vi "YokogawaInputTest.vi"() -> ()   [LabVIEW 2020]
doc: "This example shows how to measure the integrate data."
uses:
  <instrlib>/Yokogawa WT300 Series/Public/Utility/Function/Create Function String (Voltage).vi
  <instrlib>/Yokogawa WT300 Series/Public/Utility/Function/Create Function String (Current).vi
  <instrlib>/Yokogawa WT300 Series/Public/Utility/Function/Create Function String (Power).vi
  <instrlib>/Yokogawa WT300 Series/Public/Utility/Function/Create Function String (Integrate).vi
  <instrlib>/Yokogawa WT300 Series/Public/Utility/Function/Create Function String (Harmonics).vi
  <instrlib>/Yokogawa WT300 Series/Public/Data/Read Measurement (Normal).vi
  <instrlib>/Yokogawa WT300 Series/Yokogawa WT300 Series.lvlib
panel:
  out "Loop Time":u32
  in  "Reset":bool
  out "Function":string[](array[string])
  out "Measurement":dbl[](array[numeric])
  in  "Stop":bool
  in  "Update Rate (100ms)":dbl(ring)=0.1 items=["100m"=0.1, "250m"=0.25, "500m"=0.5, "1"=1.0, "2"=2.0, "5"=5.0]
  in  "Timeout (10000 ms)":i32=10000 min=1
  in  "VISA resource name":refnum<visa-resource-name>="TCPIP::192.168.1.18::INSTR"
  # "(c) 2013 Yokogawa Meters & Instruments Corporation.  All rights reserved."
  # "WT300 SERIES POWER ANALYZER"
  # "s"
  # "ms"
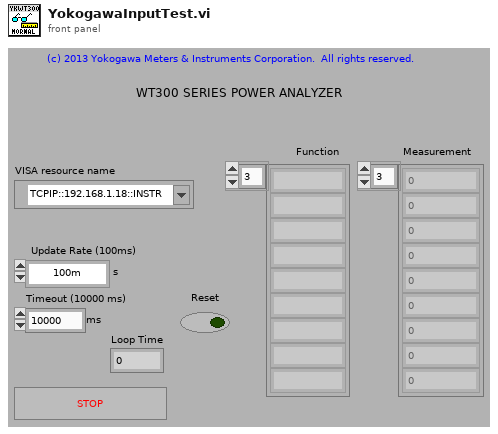
[diagram p1: front panel]
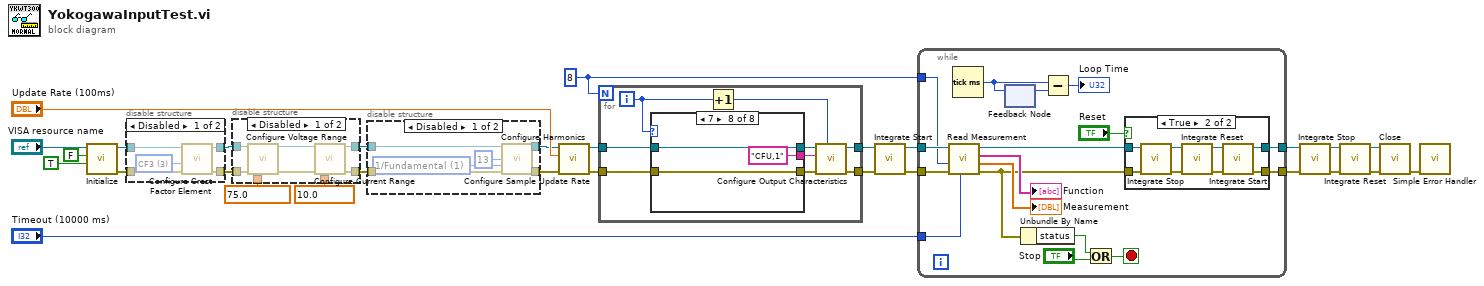
[diagram p0: block diagram]
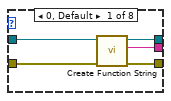
[diagram p5: hidden frame]
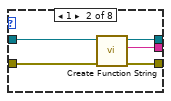
[diagram p6: hidden frame]
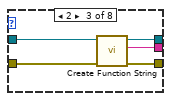
[diagram p7: hidden frame]
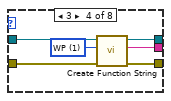
[diagram p8: hidden frame]
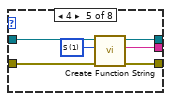
[diagram p9: hidden frame]
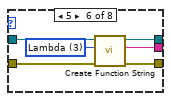
[diagram p10: hidden frame]
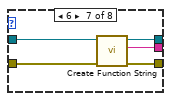
[diagram p11: hidden frame]
diagram:
  w9 = 75.0 items=["15 <7.5>"=7.5, "30 <15>"=15.0, "60 <30>"=30.0, "150 <75>"=75.0, "300 <150>"=150.0, "600 <300>"=300.0] ("Manual Range (600 <300> V)")
  w10 = 10.0 items=["5m <2.5m>"=0.0025, "10m <5m>"=0.005, "20m <10m>"=0.01, "50m <25m>"=0.025, "100m <50m>"=0.05, "200m <100m>"=0.1, "500m <250m>"=0.25, "1 <500m>"=0.5, "2 <1>"=1.0, "5 <2.5>"=2.5, "10 <5>"=5.0, "20 <10>"=10.0, "40 <20>"=20.0] ("Manual Range (20 <10> A)")
  w24 = 8
  n1 = call <instrlib>:"Initialize.vi"("Reset (True)"=TRUE ("Reset? (True)"), "ID Query (True)"=FALSE, "VISA resource name"="VISA resource name") -> ("error out"=w1:errorcluster, "VISA resource name out"=w2:refnum<visa-resource-name>)  [unwired: 7 in]
  n2 = disable-structure shown="Disabled" {
    disable-tunnel: [w34 w36] -> w11
    disable-tunnel: w2 -> [w32 w36]
    disable-tunnel: [w31 w35] -> w8
    disable-tunnel: w1 -> [w30 w35]
    frame Disabled {
      w33 = 3 items=["CF3"=3, "CF6"=6] ("Crest Factor (3: CF3)")
      n3 = call "Configure Crest Factor Element.vi"("error in (no error)"=w30, "Crest Factor (3: CF3)"=w33, "VISA resource name"=w32) -> ("error out"=w31:errorcluster, "VISA resource name out"=w34:refnum<visa-resource-name>)  [unwired: 7 in]
    }
    frame Enabled {
    }
  }
  n4 = disable-structure shown="Disabled" {
    disable-tunnel: w11 -> [w44 w46]
    disable-tunnel: w10 -> [w42 _]
    disable-tunnel: w9 -> [w41 _]
    disable-tunnel: [w40 w46] -> w6
    disable-tunnel: w8 -> [w39 w45]
    disable-tunnel: [w37 w45] -> w4
    frame Disabled {
      n5 = call "Configure Voltage Range.vi"("VISA resource name"=w44, "error in (no error)"=w39, "Manual Range (600 <300> V)"=w41) -> ("VISA resource name out"=w43:refnum<visa-resource-name>, "error out"=w38:errorcluster)  [unwired: 11 in]
      n6 = call "Configure Current Range.vi"("VISA resource name"=w43, "error in (no error)"=w38, "Manual Range (20 <10> A)"=w42) -> ("VISA resource name out"=w40:refnum<visa-resource-name>, "error out"=w37:errorcluster)  [unwired: 11 in]
    }
    frame Enabled {
    }
  }
  n7 = disable-structure shown="Disabled" {
    disable-tunnel: [w50 w54] -> w7
    disable-tunnel: w6 -> [w49 w54]
    disable-tunnel: [w48 w53] -> w5
    disable-tunnel: w4 -> [w47 w53]
    frame Disabled {
      w52 = 1 items=["1/Total", "1/Fundamental"] ("Distortion Factor (0: 1/Total)")
      n8 = call "Configure Harmonics.vi"("VISA resource name"=w49, "Maximum Order (50)"=13, "Distortion Factor (0: 1/Total)"=w52, "error in (no error)"=w47) -> ("VISA resource name out"=w50:refnum<visa-resource-name>, "error out"=w48:errorcluster)  [unwired: 10 in]
    }
    frame Enabled {
    }
  }
  n9 = call <instrlib>:"Configure Sample Update Rate.vi"("error in (no error)"=w5, "Update Rate (500m s)"="Update Rate (100ms)", "VISA resource name"=w7) -> ("error out"=w25:errorcluster, "VISA resource name out"=w26:refnum<visa-resource-name>)  [unwired: 7 in]
  n10 = for {
    N: w24 -> [_]
    tunnel: [w63] -> w14
    tunnel: [w62] -> w13
    tunnel: w26 -> [w58]
    tunnel: w25 -> [w57]
    i -> [w55]
    n11 = case shown="7" w55 {
      tunnel: [w68 w73 w78 w84 w85 w91 w101 "CFU,1" ("Function String")] -> w61
      tunnel: [w67 w72 w77 w83 w89 w95 w100 w103] -> w60
      tunnel: [w66 w71 w76 w82 w87 w93 w99 w102] -> w59
      tunnel: w58 -> [w65 w70 w75 w81 w90 w96 w98 w103]
      tunnel: w57 -> [w64 w69 w74 w80 w88 w94 w97 w102]
      frame 0, Default {
        n12 = call-poly <instrlib>:"Create Function String.vi"("error in (no error)"=w64, "VISA resource name"=w65) -> ("error out"=w66:errorcluster, "Function String"=w68:string, "VISA resource name out"=w67:refnum<visa-resource-name>)  [unwired: 7 in]
      }
      frame 1 {
        n13 = call-poly <instrlib>:"Create Function String.vi"("error in (no error)"=w69, "VISA resource name"=w70) -> ("error out"=w71:errorcluster, "Function String"=w73:string, "VISA resource name out"=w72:refnum<visa-resource-name>)  [unwired: 7 in]
      }
      frame 2 {
        n14 = call-poly <instrlib>:"Create Function String.vi"("error in (no error)"=w74, "VISA resource name"=w75) -> ("error out"=w76:errorcluster, "Function String"=w78:string, "VISA resource name out"=w77:refnum<visa-resource-name>)  [unwired: 7 in]
      }
      frame 3 {
        w79 = 1 items=["Time", "WP", "WP+", "WP-", "q", "q+", "q-", "Math"] ("Function (0: Time)")
        n15 = call-poly <instrlib>:"Create Function String.vi"("error in (no error)"=w80, "Function (0: Time)"=w79, "VISA resource name"=w81) -> ("error out"=w82:errorcluster, "Function String"=w84:string, "VISA resource name out"=w83:refnum<visa-resource-name>)  [unwired: 6 in]
      }
      frame 4 {
        w86 = 1 items=["P", "S", "Q", "Lambda", "Phi", "P+peak", "P-peak"] ("Function (0: P)")
        n16 = call-poly <instrlib>:"Create Function String.vi"("error in (no error)"=w88, "Function (0: P)"=w86, "VISA resource name"=w90) -> ("error out"=w87:errorcluster, "Function String"=w85:string, "VISA resource name out"=w89:refnum<visa-resource-name>)  [unwired: 6 in]
      }
      frame 5 {
        w92 = 3 items=["P", "S", "Q", "Lambda", "Phi", "P+peak", "P-peak"] ("Function (0: P)")
        n17 = call-poly <instrlib>:"Create Function String.vi"("error in (no error)"=w94, "Function (0: P)"=w92, "VISA resource name"=w96) -> ("error out"=w93:errorcluster, "Function String"=w91:string, "VISA resource name out"=w95:refnum<visa-resource-name>)  [unwired: 6 in]
      }
      frame 6 {
        n18 = call-poly <instrlib>:"Create Function String.vi"("error in (no error)"=w97, "VISA resource name"=w98) -> ("error out"=w99:errorcluster, "Function String"=w101:string, "VISA resource name out"=w100:refnum<visa-resource-name>)  [unwired: 7 in]
      }
      frame 7 {
      }
    }
    n19 = Increment(x=w55) -> (x+1=w56:i32)
    n20 = call <instrlib>:"Configure Output Characteristics.vi"("Item (1)"=w56, "error in (no error)"=w59, "Function (Empty)"=w61, "VISA resource name"=w60) -> ("error out"=w62:errorcluster, "VISA resource name out"=w63:refnum<visa-resource-name>)  [unwired: 6 in]
  }
  n21 = call <instrlib>:"Integrate Start.vi"("error in (no error)"=w13, "VISA resource name"=w14) -> ("error out"=w22:errorcluster, "VISA resource name out"=w23:refnum<visa-resource-name>)  [unwired: 8 in]
  n22 = while {
    tunnel: [w111] -> w21
    tunnel: [w109] -> w20
    tunnel: "Timeout (10000 ms)" -> [w121]
    tunnel: w23 -> [w120]
    tunnel: w22 -> [w119]
    tunnel: w24 -> [w118]
    stop <- w115 stop-if-true
    n23 = call-poly <instrlib>:"Read Measurement.vi"("Timeout (10000 ms)"=w121, "error in (no error)"=w119, "Number of Item (15)"=w118, "VISA resource name"=w120) -> ("error out"=w110:errorcluster, "Measurement"=→"Measurement":dbl[], "Function"=→"Function":string[], "VISA resource name out"=w112:refnum<visa-resource-name>)  [unwired: 4 in]
    n24 = Tick Count (ms)() -> (millisecond timer value=w105:u32)
    n25 = feedback #1() -> (w106:u32)  [unwired: 1 in]
    n26 = feedback-in #1(w105) -> ()
    n27 = Unbundle By Name ("名前でバンドル解除")(w110) -> ("status"=w116:bool)
    n28 = Subtract(x=w105, y=w106) -> (x-y=→"Loop Time":u32)
    n29 = Or(x=w116, y="Stop") -> (x .or. y?=w115:bool)
    n30 = case shown="True" "Reset" {
      tunnel: w112 -> [w123 w131]
      tunnel: [w123 w126] -> w111
      tunnel: w110 -> [w122 w129]
      tunnel: [w122 w124] -> w109
      frame False {
      }
      frame True {
        n31 = call <instrlib>:"Integrate Stop.vi"("error in (no error)"=w129, "VISA resource name"=w131) -> ("error out"=w128:errorcluster, "VISA resource name out"=w130:refnum<visa-resource-name>)  [unwired: 8 in]
        n32 = call <instrlib>:"Integrate Reset.vi"("error in (no error)"=w128, "VISA resource name"=w130) -> ("error out"=w125:errorcluster, "VISA resource name out"=w127:refnum<visa-resource-name>)  [unwired: 8 in]
        n33 = call <instrlib>:"Integrate Start.vi"("error in (no error)"=w125, "VISA resource name"=w127) -> ("error out"=w124:errorcluster, "VISA resource name out"=w126:refnum<visa-resource-name>)  [unwired: 8 in]
      }
    }
  }
  n34 = call <instrlib>:"Integrate Stop.vi"("error in (no error)"=w20, "VISA resource name"=w21) -> ("error out"=w16:errorcluster, "VISA resource name out"=w18:refnum<visa-resource-name>)  [unwired: 8 in]
  n35 = call <instrlib>:"Integrate Reset.vi"("error in (no error)"=w16, "VISA resource name"=w18) -> ("error out"=w15:errorcluster, "VISA resource name out"=w17:refnum<visa-resource-name>)  [unwired: 8 in]
  n36 = call <instrlib>:"Close.vi"("error in (no error)"=w15, "VISA resource name"=w17) -> ("error out"=w29:errorcluster)  [unwired: 9 in]
  n37 = call <vilib>:"Simple Error Handler.vi"("error in (no error)"=w29) -> ()  [unwired: 4 in, 5 out]
